vi "Read TOML File (TOML).vi"(8 "error in (no error)":errorcluster, 11 "file path (use dialog)":path) -> (0 "error out":errorcluster, 3 "Value":T1)   [LabVIEW 2020, in "TOML.lvlib"]
uses:
  TOML.lvlib
  TOML Value.ctl
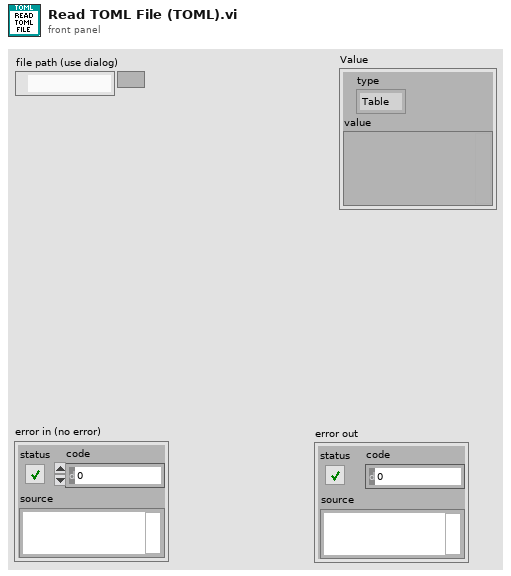
[diagram p1: front panel]
types:
  T1 = typedef "TOML.lvlib/TOML Value.ctl" = cluster{"type":enum16{"Table", "Array", "String", "Integer", "Float", "Boolean", "Offset Date-Time", "Local Date-Time", "Local Date", "Local Time", "Path"}, "value":variant}
  T2 = enum16{"open", "replace", "create", "open or create", "replace or create", "replace or create with confirmation"}
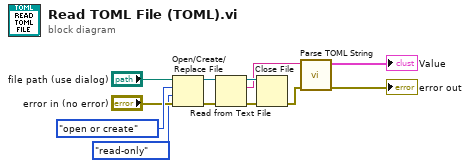
[diagram p0: block diagram]
diagram:
  n1 = Open/Create/Replace File(file path (use dialog)="file path (use dialog)", error in="error in (no error)", operation (0:open)=T2."open or create", access (0:read/write)=enum16{"read/write", "read-only", "write-only"}."read-only") -> (refnum out=w9:refnum<file>, error out=w10:errorcluster)  [unwired: 2 in, 1 out]
  n2 = Read from Text File(file (use dialog)=w9, error in=w10) -> (refnum out=w7:refnum<file>, text=w5:string, error out=w8:errorcluster)  [unwired: 2 in, 1 out]
  n3 = Close File(refnum=w7, error in=w8) -> (error out=w4:errorcluster)  [unwired: 1 out]
  n4 = call "Parse TOML String.vi"("error in (no error)"=w4, "String"=w5) -> ("error out"=→"error out":errorcluster, "Value"=→"Value":T1)  [unwired: 8 in]
